vi "FRAS Commande.vi"(0 "CdG commmande":dbl[](array[numeric]), 7 "FRAS_matrice_commande":dbl[][](array[numeric]), 11 "Nb Echantillons":i32) -> (8 "FRAS Commande":dbl[][](array[numeric]))   [LabVIEW 2020]
uses:
  <vilib>/Analysis/baseanly.llb/A x Vector.vi
  <vilib>/Analysis/Matrix/Numeric/Conversions/Array To Matrix - RA2.vi
  <vilib>/Analysis/NI_AALBase.lvlib
  <vilib>/Analysis/Matrix/NI_Matrix.lvlib
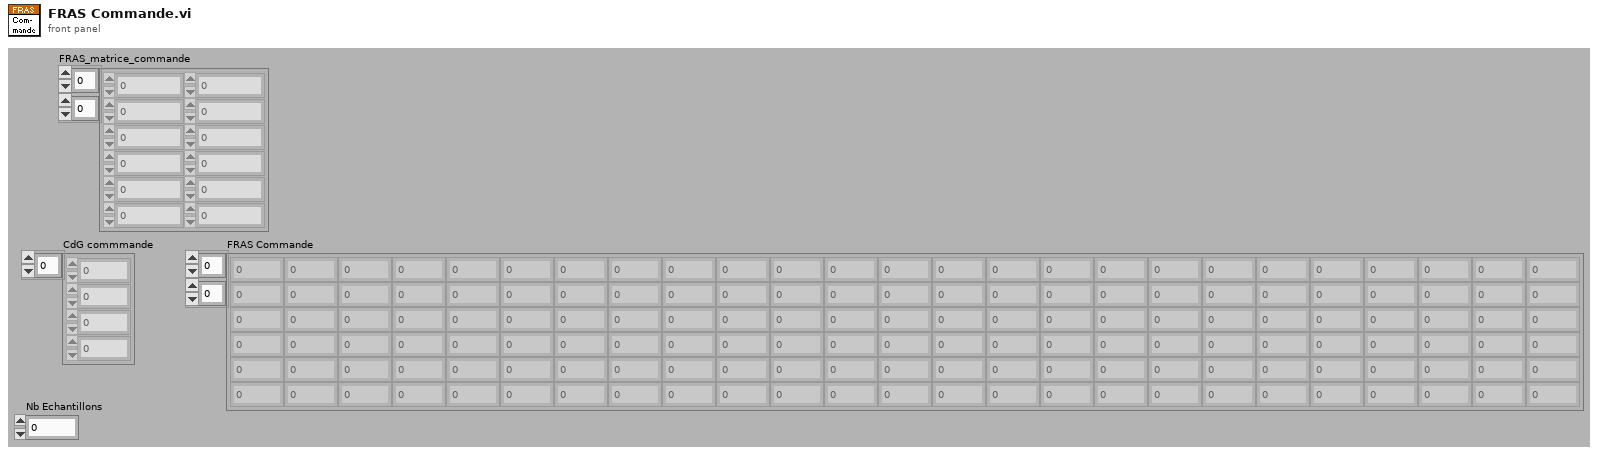
[diagram p1: front panel]
types:
  T1 = typedef "NI_Matrix.lvlib/RealMatrix.ctl" = dbl[][]
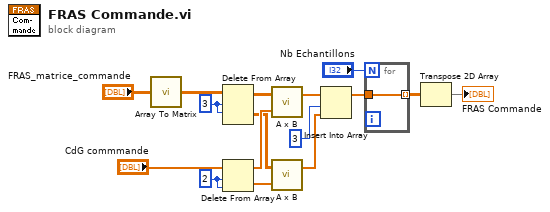
[diagram p0: block diagram]
diagram:
  w3 = 3 ("longueur")
  w12 = 2 ("longueur")
  n1 = call-poly <vilib>:"Array To Matrix.vi"("Real 2D Array"="FRAS_matrice_commande") -> ("Real Matrix"=w2:T1)
  n2 = Delete From Array(array=w2, length=w3, index (row)=w3) -> (deleted portion=w10:T1, array with subset deleted=w14:T1)  [unwired: 1 in]
  n3 = Delete From Array(array="CdG commmande", length=w12, index=w12) -> (deleted portion=w9:dbl[], array with subset deleted=w11:dbl[])
  n4 = call-poly <vilib>:"A x B.vi"("Vector"=w11, "A"=w14) -> ("A x Vector"=w8:dbl[])  [unwired: 1 out]
  n5 = call-poly <vilib>:"A x B.vi"("Vector"=w9, "A"=w10) -> ("A x Vector"=w7:dbl[])  [unwired: 1 out]
  n6 = Insert Into Array(array=w8, index=3 ("indice"), new element=w7) -> (w5:dbl[])
  n7 = for {
    N: "Nb Echantillons" -> [_]
    tunnel: w5 -> [w17]
    tunnel: [w17] -> w16 mode=indexing
  }
  n8 = Transpose 2D Array(2D array=w16) -> (transposed array=→"FRAS Commande":dbl[][])
